vi "FGGA Serial Data Server & Recordingv4.2.vi"() -> ()   [LabVIEW 2014]
uses:
  <vilib>/Instr/_visa.llb/VISA Set IO Buffer Mask.ctl
  <vilib>/Instr/_visa.llb/VISA Flush IO Buffer Mask.ctl
  <vilib>/Platform/TimedLoop/XDataNode/timing_clust.ctl
  <vilib>/Platform/TimedLoop/XDataNode/nitl_modes.ctl
  <vilib>/Platform/TimedLoop/XDataNode/wakeup.ctl
  C:/Program Files (x86)/National Instruments/LabVIEW 2014/examples/Data Communication/Network Streams/Simple Network Streams/support/Network Stream Command.ctl
  <vilib>/Utility/error.llb/whitespace.ctl
  <vilib>/Instr/_visa.llb/VISA Configure Serial Port (Instr).vi
  <vilib>/Utility/tcp.llb/UDP Multicast Write-Only Open.vi
  <vilib>/platform/TimedLoop/XDataNode/XDataNode.xnode
  <vilib>/Platform/TimedLoop/XDataNode/XDNodeRunTimeDep.lvlib
panel:
  out "FGGA Pump":bool
  out "Flight Number":string
  out "Stop File Write":bool
  out "Default file name":string
  out "MFC":dbl[](array[numeric])
  out "FGGA restart":bool
  out "V4":bool
  out "V3":bool
  out "V2":bool
  out "V1":bool
  out "error out 2":errorcluster
  out "error out":errorcluster
  in  "MFC_1 SLPM set value":dbl
  out "Value Read":string
  out "status":bool
  in  "VISA resource name":refnum<visa-resource-name>="ASRL3::INSTR"
  in  "timeout (10sec) 2":u32=3000
  out "Labview_Viewer_UDP_Error_Out":errorcluster
  in  "Clear Display\nErrors":bool
  out "Data Processing":bool
  out "TCP Binary Packet":string
  out "UDP Time Stamp Offset":i32=1
  out "Data String":string
  out "UDP_ACSII_Out":string
  out "Serial error out":errorcluster
  out "SEPTIC TCP Error Out":errorcluster
  out "TCP packet\nSend To SEPTIC":bool
  out "FISH TCP Error Out":errorcluster
  out "TCP packet\nSend To FISH":bool
  out "UDP_Pack_num":u32
  out "UDP_Out Status":bool
  out "UDP_Out_Error Out":errorcluster
  out "Data Array":string[](array[string])
  out "RAW DATA":string
  in  "stop":bool
  in  "timeout (10sec)":u32=1500
  in  "VISA resource name":refnum<visa-resource-name>="ASRL7::INSTR"
  out "Number of times \nRead time out":u32
  out "Loop count":i32
  # "Date"
  # "Time"
  # "CH4"
  # "CO2"
  # "H2O"
  # "Cell Pressure"
  # "Cell Temperature"
  # "Spectral Flag"
  # "Ring Down Time (Laser A)"
  # "Ring Down Time (Laser B)"
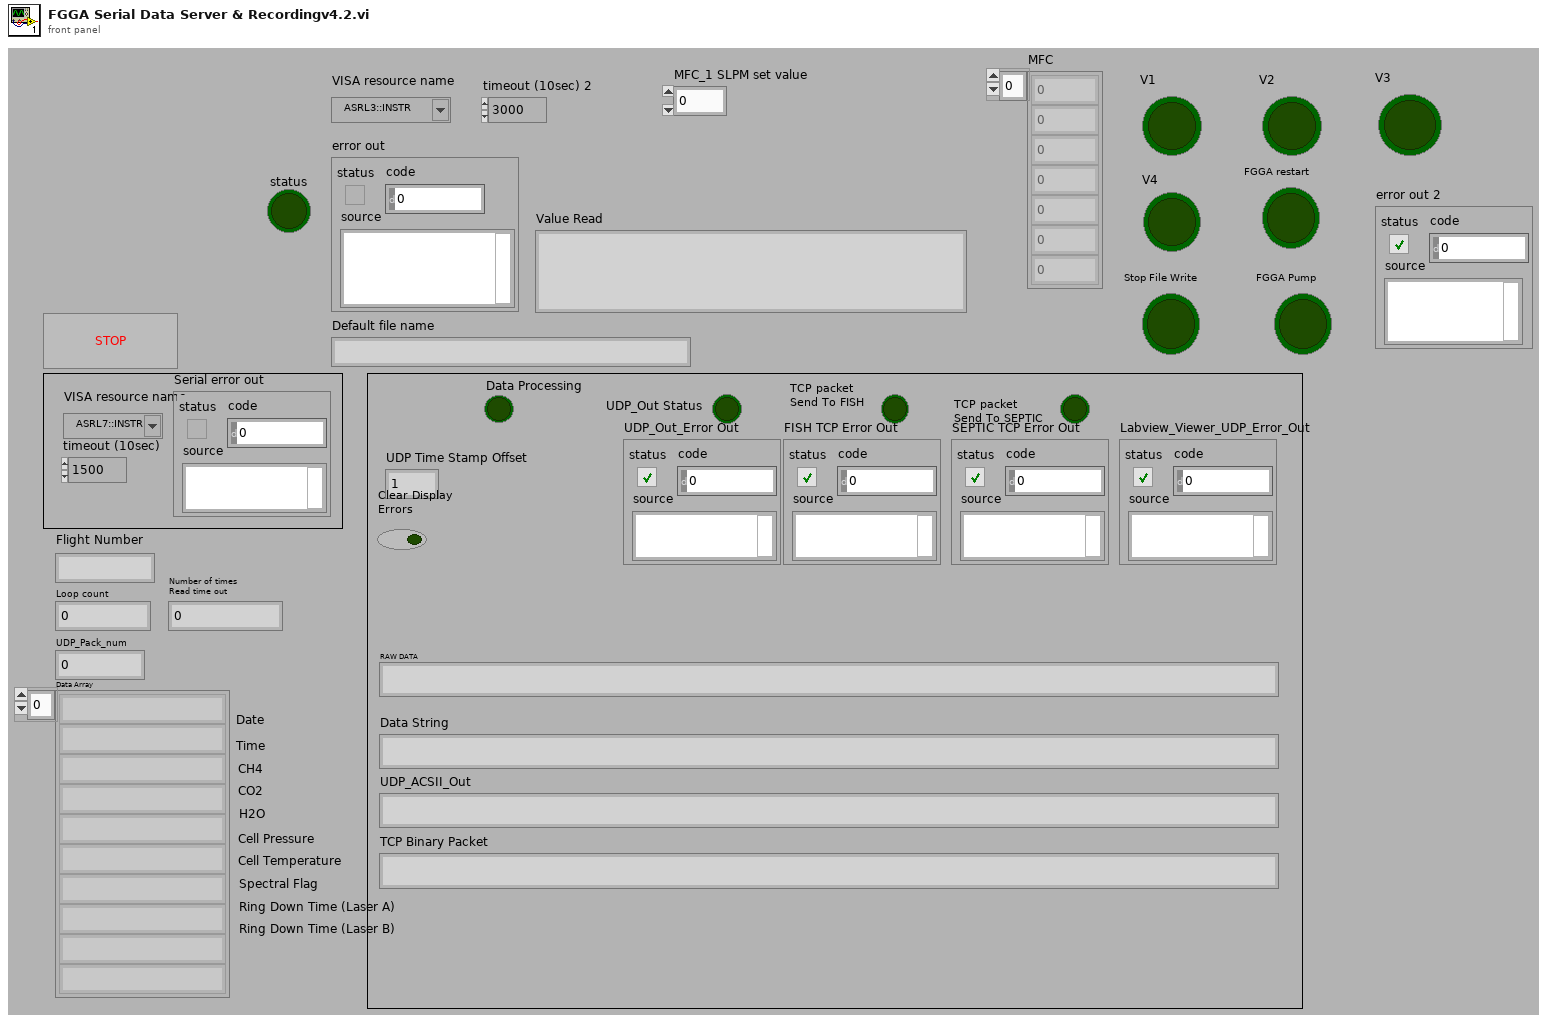
[diagram p1: front panel]
types:
  T1 = typedef "VISA Flush IO Buffer Mask.ctl" = u16
  T2 = typedef "VISA Set IO Buffer Mask.ctl" = u16
  T3 = typedef "XDNodeRunTimeDep.lvlib/timing_clust.ctl" = cluster{"Expected End [f-1]":u64, "Actual End [f-1]":u64, "Finished Late? [f-1]":bool, "Expected End [i-1]":u64, "Actual End [i-1]":u64, "Finished Late? [i-1]":bool, "Expected Start [i]":u64, "Actual Start [i]":u64, "Expected Start [f]":u64, "Actual Start [f]":u64, "Source Name":string, "Structure Name":string, "Period":i64, "Deadline":i64, "Offset":i64, "Start":i64, "Priority":i32, "Timeout":i32, "Mode":T4, "Wakeup Reason":T5, "Error":errorcluster, "Source Type":string, "Secondary Source Type":string, "Global End Time":u64, "Global Start Time":u64, "Frame Duration":u64, "Iteration Duration":u64, "Assigned CPU":i32, "I/O Scan Engine Mode":u32}
  T4 = typedef "XDNodeRunTimeDep.lvlib/nitl_modes.ctl" = enum32{"No Change", "Process missed periods, maintain original phase", "Discard missed periods, maintain original phase", "Process missed periods, ignore original phase", "Discard missed periods, ignore original phase"}
  T5 = typedef "XDNodeRunTimeDep.lvlib/wakeup.ctl" = enum32{"Normal", "Aborted", "Asynchronous wakeup", "Timing source error", "Timed loop error", "Timeout"}
  T6 = typedef "Network Stream Command.ctl" = cluster{"Message":string, "Message Data":variant}
  T7 = enum16{"open", "replace", "create", "open or create", "replace or create", "replace or create with confirmation"}
  T8 = typedef "whitespace.ctl" = u16
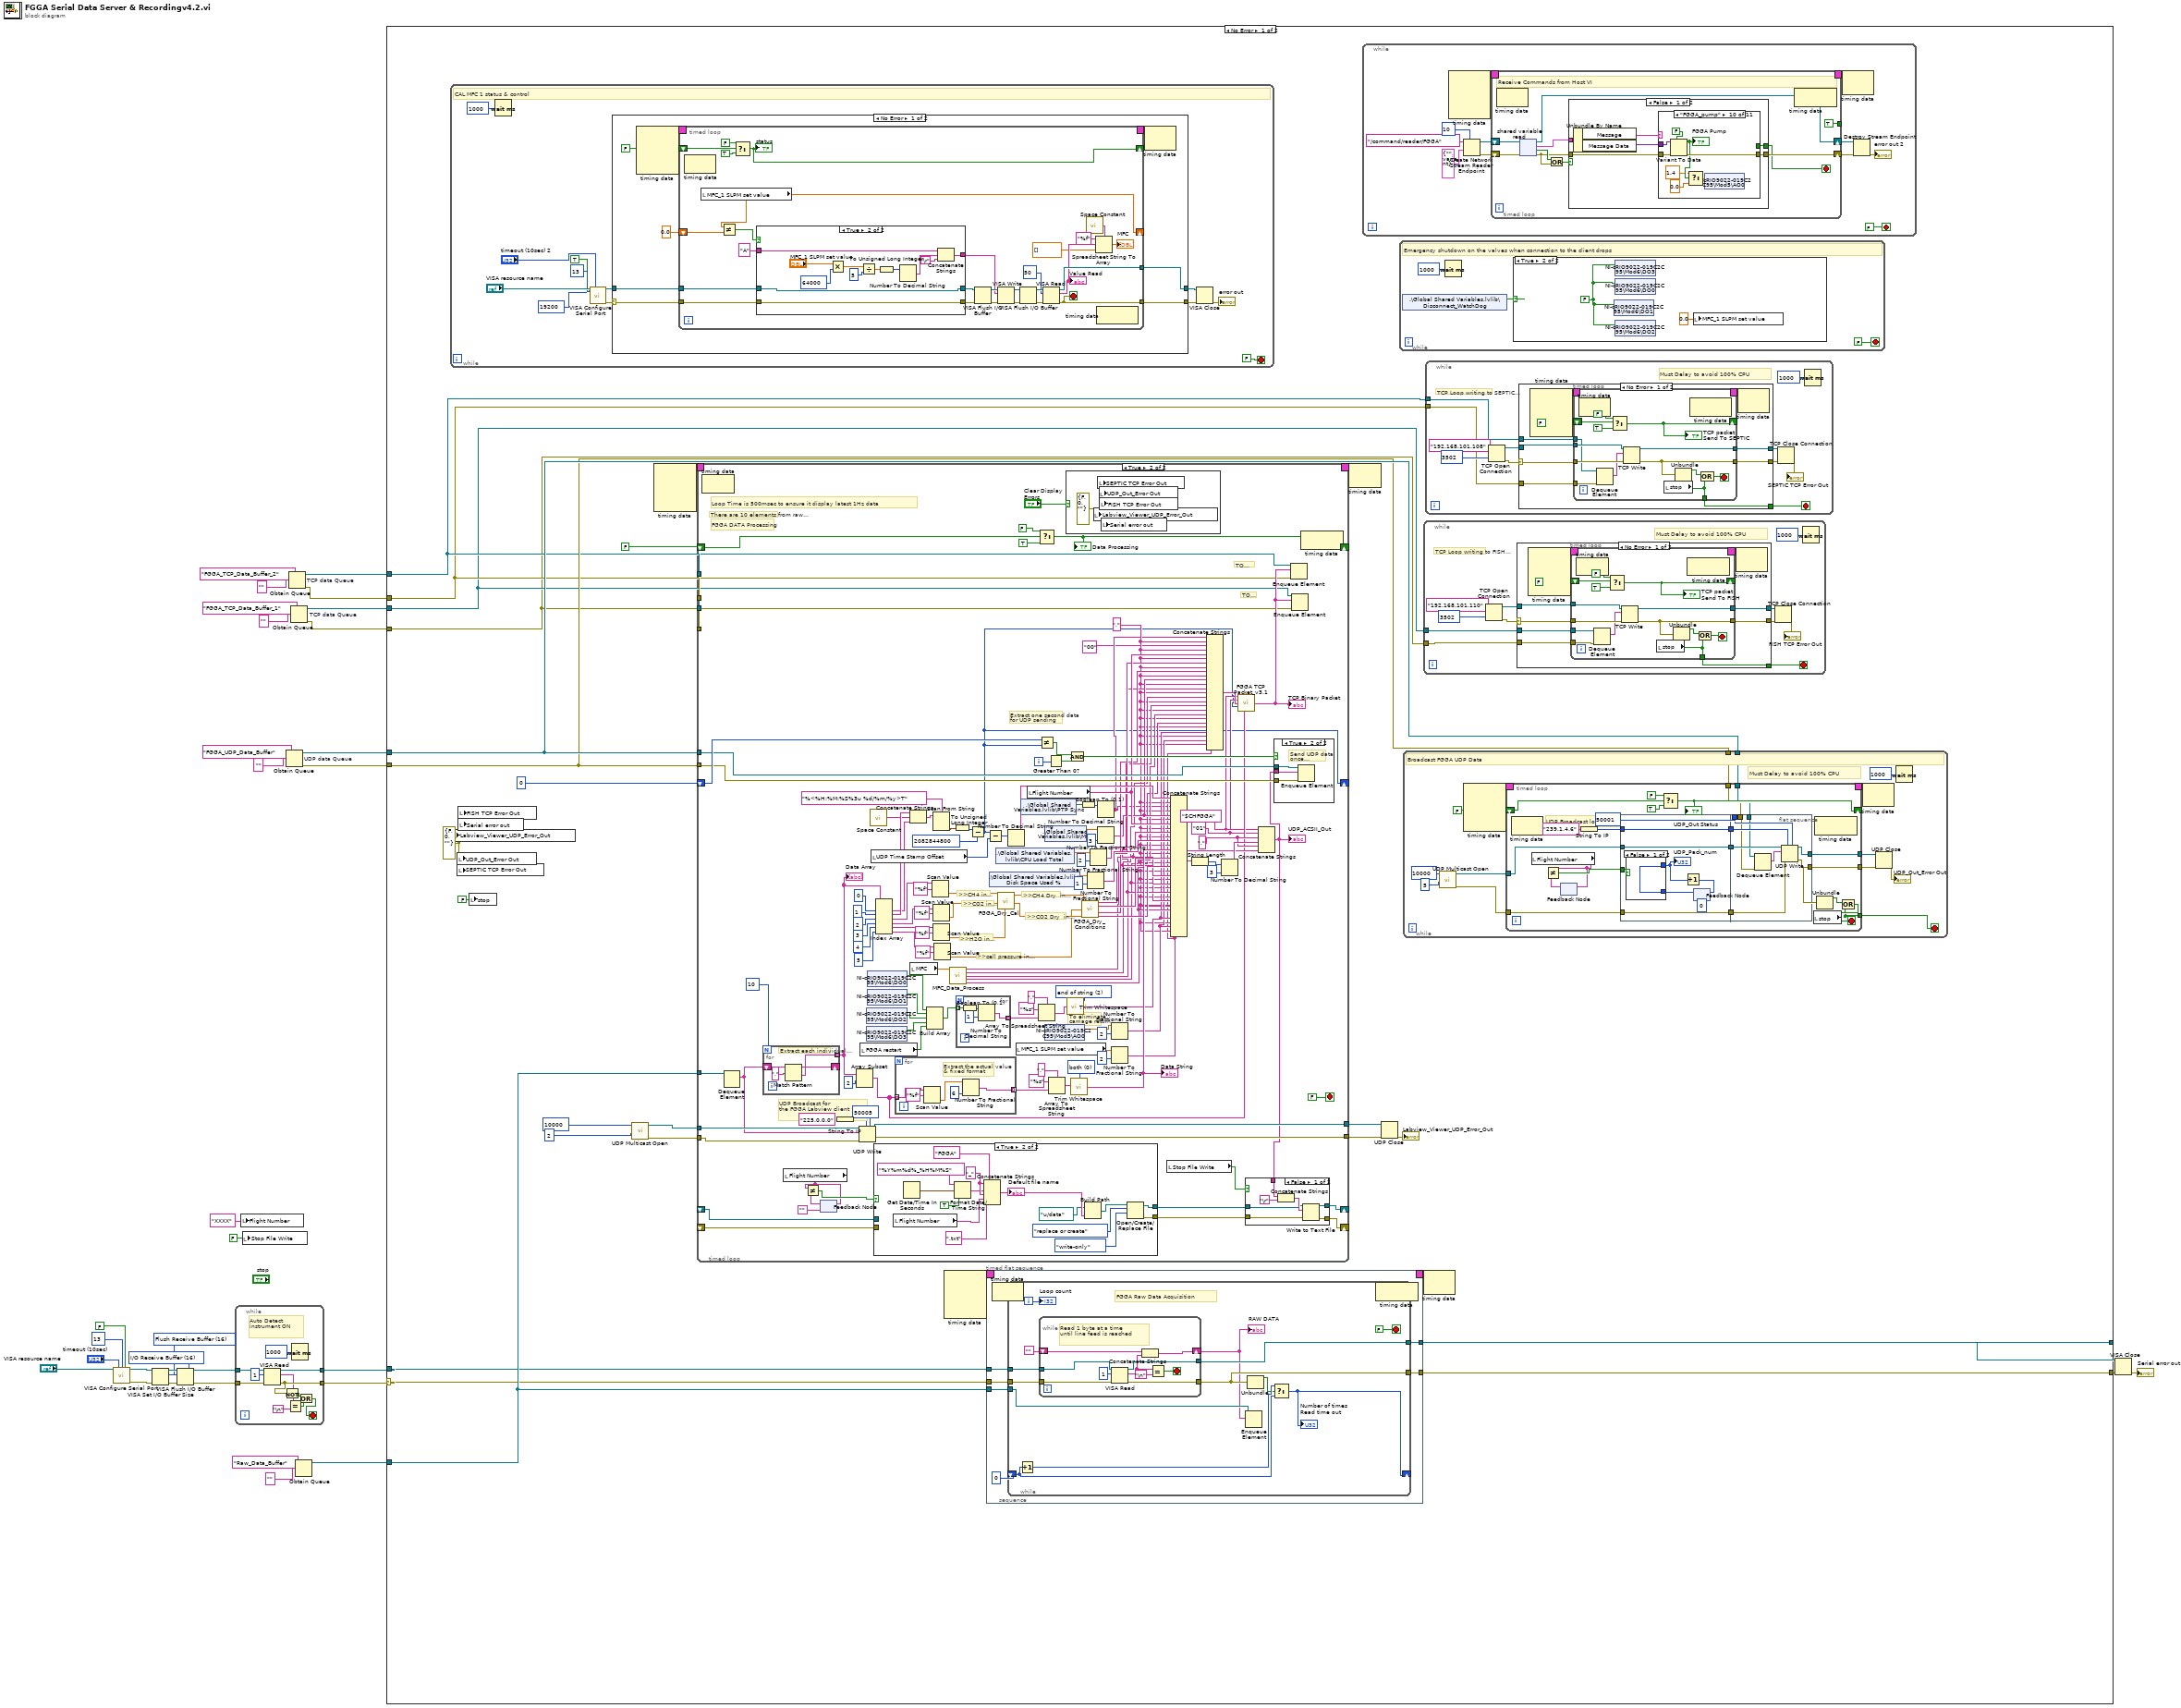
[diagram p0: block diagram]
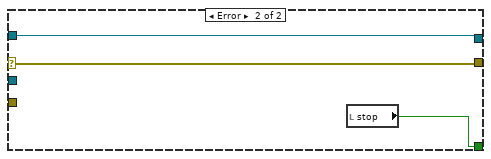
[diagram p3: hidden frame]
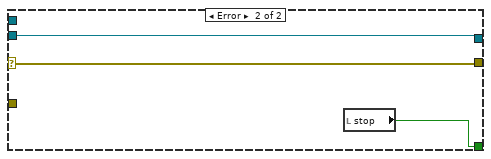
[diagram p4: hidden frame]
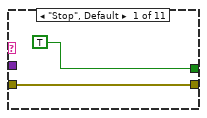
[diagram p5: hidden frame]
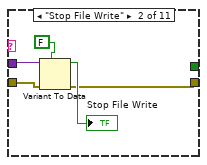
[diagram p6: hidden frame]
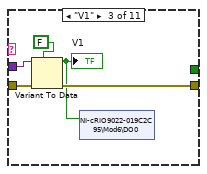
[diagram p7: hidden frame]
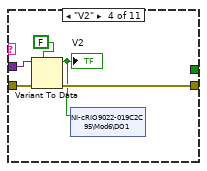
[diagram p8: hidden frame]
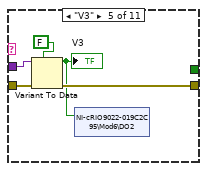
[diagram p9: hidden frame]
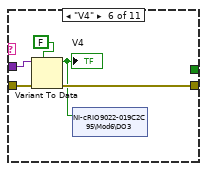
[diagram p10: hidden frame]
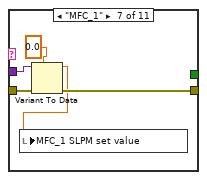
[diagram p11: hidden frame]
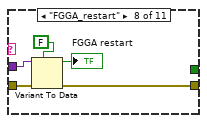
[diagram p12: hidden frame]
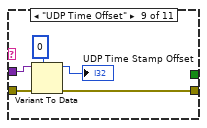
[diagram p13: hidden frame]
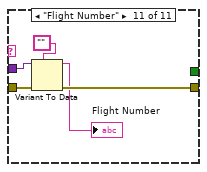
[diagram p14: hidden frame]
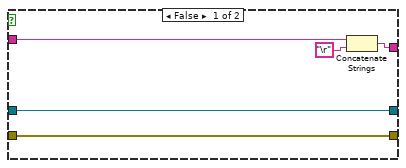
[diagram p16: hidden frame]
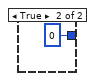
[diagram p18: hidden frame]
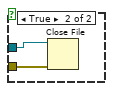
[diagram p20: hidden frame]
diagram:
  w9 = T1 16 items=["Flush Receive Buffer"=16, "Write Transmit Buffer to Device"=32, "Flush Receive Buffer (No I/O)"=64, "Flush Transmit Buffer"=128] ("Mask")
  w10 = T2 16 items=["I/O Receive Buffer"=16, "I/O Transmit Buffer"=32, "I/O Receive and Transmit Buffer"=48] ("Mask")
  n1 = call-poly "VISA Configure Serial Port"("VISA resource name"="VISA resource name", "timeout (10sec)"="timeout (10sec)", "termination char\n(0xA = '\\n' = LF)"=u8 13 ("termination char\n(0xA = '\\n' = LF)"), "Enable Termination\nChar (T)"=FALSE ("Enable Termination\nChar (T)")) -> ("VISA resource name out"=w8:refnum<visa-resource-name>, "error out"=w7:errorcluster)  [unwired: 10 in]
  n2 = VISA Set I/O Buffer Size(VISA resource name=w8, mask (16)=w10, error in (no error)=w7) -> (VISA resource name out=w11:refnum<visa-resource-name>, error out=w12:errorcluster)  [unwired: 1 in]
  n3 = VISA Flush I/O Buffer(VISA resource name=w11, mask (16)=w9, error in (no error)=w12) -> (VISA resource name out=w6:refnum<visa-resource-name>, error out=w5:errorcluster)
  n4 = while {
    tunnel: w6 -> [w45]
    tunnel: w5 -> [w44]
    tunnel: [w42] -> w4
    tunnel: [w41] -> w3
    stop <- w36 stop-if-true
    # "Auto Detect\ninstrument ON"
    n5 = VISA Read(VISA resource name=w45, byte count=u32 1, error in (no error)=w44) -> (VISA resource name out=w41:refnum<visa-resource-name>, read buffer=w39:string, error out=w42:errorcluster)  [unwired: 1 out]
    n6 = Not(x=w42) -> (.not. x?=w38:bool)
    n7 = Equal?(x=w39, y="\n") -> (x = y?=w37:bool)
    n8 = Wait (ms)(milliseconds to wait=u32 1000) -> ()  [unwired: 1 out]
    n9 = Or(x=w38, y=w37) -> (x .or. y?=w36:bool)
  }
  n10 = local write "Flight Number"("XXXX" ("Flight Number")) -> ()
  n11 = local write "Stop File Write"(FALSE ("Stop File Write")) -> ()
  n12 = Obtain Queue "UDP data Queue"(name (unnamed)="FGGA_UDP_Data_Buffer", element data type="") -> (queue out=w22:refnum<queue>, error out=w21:errorcluster)  [unwired: 3 in, 1 out]
  n13 = Obtain Queue "TCP data Queue"(name (unnamed)="FGGA_TCP_Data_Buffer_2", element data type="") -> (queue out=w16:refnum<queue>, error out=w15:errorcluster)  [unwired: 3 in, 1 out]
  n14 = Obtain Queue "TCP data Queue"(name (unnamed)="FGGA_TCP_Data_Buffer_1", element data type="") -> (queue out=w14:refnum<queue>, error out=w13:errorcluster)  [unwired: 3 in, 1 out]
  n15 = Obtain Queue(name (unnamed)="Raw_Data_Buffer", element data type="") -> (queue out=w28:refnum<queue>)  [unwired: 3 in, 2 out]
  n16 = case shown="No Error" w4 {
    selector: w4 -> [w48 w595]
    tunnel: w3 -> [w49 w596]
    tunnel: [w70 w596] -> w25
    tunnel: [w71 w595] -> w26
    tunnel: w28 -> [w67 _]
    tunnel: w22 -> [w65 _]
    tunnel: w21 -> [w64 _]
    tunnel: w16 -> [w63 _]
    tunnel: w15 -> [w62 _]
    tunnel: w14 -> [w61 _]
    tunnel: w13 -> [w60 _]
    frame No Error {
      w51 = errorcluster {"status"=FALSE, "code"=0, "source"=""} ("UDP Error Out")
      n17 = while {
        stop <- FALSE stop-if-true
        # "CAL MFC 1 status & control"
        n18 = Wait (ms)(milliseconds to wait=u32 1000) -> ()  [unwired: 1 out]
        n19 = call-poly "VISA Configure Serial Port"("VISA resource name"="VISA resource name", "timeout (10sec)"="timeout (10sec) 2", "termination char\n(0xA = '\\n' = LF)"=u8 13 ("termination char\n(0xA = '\\n' = LF)"), "Enable Termination\nChar (T)"=TRUE ("Enable Termination\nChar (T)"), "baud rate (9600)"=u32 19200) -> ("VISA resource name out"=w298:refnum<visa-resource-name>, "error out"=w294:errorcluster)  [unwired: 9 in]
        n20 = case shown="No Error" w294 {
          selector: w294 -> [w305 w355]
          tunnel: w298 -> [w306 w356]
          tunnel: [w304 w356] -> w297
          tunnel: [w303 w355] -> w296
          frame No Error {
            n21 = node-c288() -> (w301:T3)  [unwired: 4 in]
            n22 = timed-loop {
              tunnel: w306 -> [w329]
              tunnel: w305 -> [w327]
              tunnel: [w320] -> w304
              tunnel: [w315] -> w303
              shift-right: [w316] -> _
              shift-left: FALSE -> [w319]
              timing: w301 -> [_]
              timing-out: [_] -> w300
              shift-right: [w307] -> _
              shift-left: 0.0 -> [w309]
              stop <- w315 stop-if-true
              n23 = node-c288() -> ()  [unwired: 1 in, 1 out]
              n24 = local read "MFC_1 SLPM set value"() -> (w307:dbl)
              n25 = Not Equal?(x=w307, y=w309) -> (x != y?=w308:bool)
              n26 = Select(t=FALSE, s=w319, f=TRUE) -> (s? t:f=w316:bool)
              "status" <- w316
              n27 = case shown="True" w308 {
                tunnel: w329 -> [w337 w352]
                tunnel: [w337 w352] -> w328
                tunnel: w327 -> [w336 w351]
                tunnel: [w336 w351] -> w326
                tunnel: "A" -> [w340 w344]
                tunnel: [w338 w341] -> w324
                frame False {
                  n28 = Concatenate Strings(w340, "\r") -> (w338:string)
                }
                frame True {
                  n29 = Multiply(x="MFC_1 SLPM set value", y=u32 64000) -> (x*y=w348:dbl)
                  n30 = Divide(x=w348, y=u32 5) -> (x/y=w346:dbl)
                  n31 = To Unsigned Long Integer(number=w346) -> (unsigned 32bit integer=w345:u32)
                  n32 = Number To Decimal String(number=w345) -> (decimal integer string=w343:string)  [unwired: 1 in]
                  n33 = Concatenate Strings(w344, w343, "\r") -> (w341:string)
                }
              }
              n34 = VISA Flush I/O Buffer(VISA resource name=w328, error in (no error)=w326) -> (VISA resource name out=w331:refnum<visa-resource-name>, error out=w330:errorcluster)  [unwired: 1 in]
              n35 = VISA Write(VISA resource name=w331, write buffer=w324, error in (no error)=w330) -> (VISA resource name out=w323:refnum<visa-resource-name>, error out=w322:errorcluster)  [unwired: 1 out]
              n36 = VISA Flush I/O Buffer(VISA resource name=w323, error in (no error)=w322) -> (VISA resource name out=w333:refnum<visa-resource-name>, error out=w332:errorcluster)  [unwired: 1 in]
              n37 = VISA Read(VISA resource name=w333, byte count=u32 50, error in (no error)=w332) -> (VISA resource name out=w320:refnum<visa-resource-name>, read buffer=w314:string, error out=w315:errorcluster)  [unwired: 1 out]
              "Value Read" <- w314
              n38 = call <vilib>:"Space Constant.vi"() -> ("String"=w313:string)
              n39 = Spreadsheet String To Array(delimiter (Tab)=w313, format string="%f", spreadsheet string=w314, array type (2D Dbl)=dbl[] []) -> (array=→"MFC":dbl[])
              n40 = node-c288() -> ()  [unwired: 1 in, 1 out]
            }
            n41 = node-c288(w300) -> ()  [unwired: 1 out]
          }
          frame Error {
          }
        }
        n42 = VISA Close(VISA resource name=w297, error in (no error)=w296) -> (error out=→"error out":errorcluster)
      }
      n43 = local write "Labview_Viewer_UDP_Error_Out"(w51) -> ()
      n44 = local write "UDP_Out_Error Out"(w51) -> ()
      n45 = local write "SEPTIC TCP Error Out"(w51) -> ()
      n46 = local write "FISH TCP Error Out"(w51) -> ()
      n47 = local write "Serial error out"(w51) -> ()
      n48 = local write "stop"(FALSE ("stop")) -> ()
      n49 = call-poly <vilib>:"UDP Multicast Open.vi"("time-to-live (1)"=u16 2, "port"=u16 10000) -> ("error out"=w55:errorcluster, "connection ID"=w56:refnum<k16>)  [unwired: 8 in]
      n50 = node-c288() -> (w69:T3)  [unwired: 4 in]
      n51 = timed-loop {
        timing: w69 -> [_]
        timing-out: [_] -> w68
        tunnel: w67 -> [w547]
        tunnel: w65 -> [w503]
        tunnel: w64 -> [w502]
        shift-right: [w416] -> _
        shift-left: u32 0 -> [w506]
        tunnel: w63 -> [w499]
        tunnel: w62 -> [w498]
        tunnel: w61 -> [w497]
        tunnel: w60 -> [w496]
        shift-right: [w492] -> _
        shift-left: FALSE -> [w495]
        tunnel: w56 -> [w488]
        tunnel: w55 -> [w487]
        tunnel: [w486] -> w54
        tunnel: [w485] -> w53
        shift-right: [w472] -> _
        shift-left: _ -> [w464]
        shift-right: [w462] -> _
        shift-left: _ -> [w463]
        i -> [w505]
        stop <- FALSE stop-if-true
        w436 = T8 2 items=["both", "start of string", "end of string"] ("location (both)")
        w423 = ","
        w533 = T8 0 items=["both", "start of string", "end of string"] ("location (both)")
        w541 = ","
        w417 = "01"
        w418 = "$CHFGGA"
        # "To eliminate\ncarriage return"
        # ">>cell pressure in torr>>"
        # "UDP Broadcast for\nthe FGGA Labview client"
        # "There are 10 elements from raw packet"
        # "TO SEPTIC"
        # "TO FISH"
        # "Extract one second data\nfor UDP sending"
        # ">>CO2 Dry  in ppm>>"
        # ">>CH4 Dry  in ppb>>"
        # ">>H2O in ppm>>"
        # ">>CO2 in ppm>>"
        # ">>CH4 in ppm>>"
        # "Loop Time is 500msec to ensure it display latest 1Hz data"
        # "FGGA DATA Processing"
        n52 = node-c288() -> ()  [unwired: 1 in, 1 out]
        n53 = Dequeue Element(queue=w547) -> (element=w484:string)  [unwired: 2 in, 3 out]
        n54 = for {
          N: 10 -> [_]
          shift-right: [w589] -> _
          shift-left: w484 -> [w587]
          tunnel: [w588] -> w538 mode=indexing
          # "Extract each individual param"
          n55 = Match Pattern(string=w587, regular expression=",") -> (before substring=w588:string, after substring=w589:string)  [unwired: 1 in, 2 out]
        }
        "Data Array" <- w538
        n56 = local read "Flight Number"() -> (w461:string)
        n57 = feedback #1("" ("Flight Number")) -> (w469:string)
        n58 = Not Equal?(x=w461, y=w469) -> (x != y?=w467:bool)
        n59 = feedback-in #1(w461) -> ()
        n60 = String To IP(1:"225.0.0.0" ("name")) -> (0:w489:u32)
        n61 = Array Subset(array=w538, index=2) -> (w501:string[])  [unwired: 1 in]
        n62 = UDP Write(address=w489, port or service name=u16 50005, connection ID=w488, data in=w484, 8:w487) -> (error out=w485:errorcluster, 3:w486:refnum<k16>)  [unwired: 1 in]
        n63 = local read "FGGA restart"() -> (w446:bool)
        n64 = shared-variable "NI-cRIO9022-019C2C95\\Mod6\\DO2"() -> (w452:bool)  [unwired: 1 in, 1 out]
        n65 = shared-variable "NI-cRIO9022-019C2C95\\Mod6\\DO3"() -> (w451:bool)  [unwired: 1 in, 1 out]
        n66 = shared-variable "NI-cRIO9022-019C2C95\\Mod6\\DO0"() -> (w454:bool)  [unwired: 1 in, 1 out]
        n67 = shared-variable "NI-cRIO9022-019C2C95\\Mod6\\DO1"() -> (w453:bool)  [unwired: 1 in, 1 out]
        n68 = call <vilib>:"Space Constant.vi"() -> ("String"=w516:string)
        n69 = local read "UDP Time Stamp Offset"() -> (w435:i32)
        n70 = case shown="True" w467 {
          tunnel: [w553 w555] -> w466
          tunnel: [w552 w554] -> w465
          tunnel: w464 -> [w553 _]
          tunnel: w463 -> [w552 _]
          frame False {
          }
          frame True {
            w561 = "_" ("string")
            n71 = local read "Flight Number"() -> (w568:string)
            n72 = Get Date/Time In Seconds() -> (seconds since 1Jan1904=w556:timestamp)
            n73 = Format Date/Time String(time format string (%c)="%Y%m%d%_%H%M%S", seconds (now)=w556, UTC format=TRUE) -> (date/time string=w558:string)
            n74 = Concatenate Strings("FGGA" ("string"), w561, w558, w561, w568, ".txt" ("string")) -> (w563:string)
            "Default file name" <- w563
            n75 = Build Path(base path=path "u:/data", name or relative path=w563) -> (appended path=w567:path)
            n76 = Open/Create/Replace File(file path (use dialog)=w567, operation (0:open)=T7."replace or create", access (0:read/write)=enum16{"read/write", "read-only", "write-only"}."write-only") -> (refnum out=w555:refnum<file>, error out=w554:errorcluster)  [unwired: 3 in, 1 out]
          }
        }
        n77 = Index Array(array=w538, index #1=0 ("index"), index #2=1 ("index"), index #3=2 ("index"), index #4=3 ("index"), index #5=4 ("index"), index #6=5 ("index")) -> (element #1=w515:string, element #2=w517:string, element #3=w521:string, element #4=w520:string, element #5=w519:string, element #6=w477:string)
        n78 = for {
          tunnel: w501 -> [w585] mode=indexing
          tunnel: [w582] -> w531 mode=indexing
          # "Extract the actual value\n& fixed format"
          n79 = Scan Value(string=w585, format string="%f") -> (value=w583:dbl)  [unwired: 1 in, 1 out]
          n80 = Number To Fractional String(number=w583, precision (6)=i16 6) -> (F-format string=w582:string)  [unwired: 2 in]
        }
        n81 = Concatenate Strings(w517, w516, w515) -> (w514:string)
        n82 = local read "MFC"() -> (w473:dbl[])
        n83 = Build Array(w454, w453, w452, w451, w446) -> (w450:bool[])
        n84 = Scan Value(string=w521, format string="%f") -> (value=w523:dbl)  [unwired: 1 in, 1 out]
        n85 = Scan Value(string=w520, format string="%f") -> (value=w522:dbl)  [unwired: 1 in, 1 out]
        n86 = Scan From String(format string="%<%H:%M:%S%3u %d/%m/%y>T", input string=w514) -> (output 1=w511:timestamp)  [unwired: 3 in, 3 out]
        n87 = Scan Value(string=w519, format string="%f") -> (value=w474:dbl)  [unwired: 1 in, 1 out]
        n88 = Scan Value(string=w477, format string="%f") -> (value=w475:dbl)  [unwired: 1 in, 1 out]
        n89 = call "MFC_Data_Process.vi"("MFC"=w473) -> ("MFC Absolute Pressure"=w430:string, "MFC Temperature"=w429:string, "MFC Volumetric Flow"=w428:string, "MFC Mass Flow"=w427:string, "MFC Set Point"=w426:string)  [unwired: 10 in]
        n90 = To Unsigned Long Integer(number=w511) -> (unsigned 32bit integer=w512:u32)
        n91 = for {
          tunnel: w450 -> [w550] mode=indexing
          tunnel: [w549] -> w447 mode=indexing
          n92 = Boolean To (0,1)(Boolean=w550) -> (0, 1=w551:i16)
          n93 = Number To Decimal String(number=w551, width (-)=i16 1) -> (decimal integer string=w549:string)
        }
        n94 = Subtract(x=w512, y=u32 2082844800) -> (x-y=w416:u32)
        n95 = Subtract(x=w416, y=w435) -> (x-y=w509:u32)
        n96 = shared-variable ".\\Global Shared Variables.lvlib\\Disk Space Used %"() -> (w439:dbl)  [unwired: 1 in, 1 out]
        n97 = shared-variable ".\\Global Shared Variables.lvlib\\CPU Load Total"() -> (w460:dbl)  [unwired: 1 in, 1 out]
        n98 = call "FGGA_Dry_Cal.vi"("H2O"=w474, "CO2_Wet"=w522, "CH4_Wet"=w523) -> ("CO2_Dry"=w479:dbl, "CH4_Dry"=w481:dbl)  [unwired: 7 in]
        n99 = Number To Decimal String(number=w509) -> (decimal integer string=w510:string)  [unwired: 1 in]
        n100 = local read "MFC_1 SLPM set value"() -> (w442:dbl)
        n101 = shared-variable ".\\Global Shared Variables.lvlib\\PTP Sync"() -> (w455:bool)  [unwired: 1 in, 1 out]
        n102 = local read "Flight Number"() -> (w434:string)
        n103 = Array To Spreadsheet String(delimiter (Tab)=",", array=w447, 3:"%s" ("format string")) -> (spreadsheet string=w437:string)
        n104 = Select(t=FALSE, s=w495, f=TRUE) -> (s? t:f=w492:bool)
        "Data Processing" <- w492
        n105 = Not Equal?(x=w506, y=w416) -> (x != y?=w507:bool)
        n106 = shared-variable ".\\Global Shared Variables.lvlib\\MFM"() -> (w458:dbl)  [unwired: 1 in, 1 out]
        n107 = shared-variable "NI-cRIO9022-019C2C95\\Mod5\\AO0"() -> (w444:dbl)  [unwired: 1 in, 1 out]
        n108 = Greater Than 0?(x=w505) -> (x > 0?=w508:bool)
        n109 = Array To Spreadsheet String(delimiter (Tab)=",", array=w531, 3:"%s" ("format string")) -> (spreadsheet string=w532:string)
        n110 = case shown="True" "Clear Display\nErrors" {
          frame False {
          }
          frame True {
            w578 = errorcluster {"status"=FALSE, "code"=0, "source"=""} ("UDP Error Out")
            n111 = local write "Labview_Viewer_UDP_Error_Out"(w578) -> ()
            n112 = local write "SEPTIC TCP Error Out"(w578) -> ()
            n113 = local write "UDP_Out_Error Out"(w578) -> ()
            n114 = local write "FISH TCP Error Out"(w578) -> ()
            n115 = local write "Serial error out"(w578) -> ()
          }
        }
        n116 = call <vilib>:"Trim Whitespace.vi"("string"=w437, "location (both)"=w436) -> ("trimmed string"=w425:string)
        n117 = call <vilib>:"Trim Whitespace.vi"("string"=w532, "location (both)"=w533) -> ("trimmed string"=w530:string)
        "Data String" <- w530
        n118 = Compound Arithmetic op=AND(w507, w508) -> (w504:bool)
        n119 = Boolean To (0,1)(Boolean=w455) -> (0, 1=w456:i16)
        n120 = call "FGGA_Dry_Conditions.vi"("CH4_Dry"=w481, "Pressure"=w475, "CO2_Dry"=w479) -> ("CH4_Dry_TCP"=w433:string, "CH4_Dry_UDP"=w483:string, "CO2_Dry_TCP"=w432:string, "CO2_Dry_UDP"=w482:string)  [unwired: 9 in]
        n121 = Number To Fractional String(number=w439, precision (6)=i16 1) -> (F-format string=w438:string)  [unwired: 2 in]
        n122 = Number To Fractional String(number=w460, precision (6)=i16 2) -> (F-format string=w441:string)  [unwired: 2 in]
        n123 = Number To Decimal String(number=w456) -> (decimal integer string=w420:string)  [unwired: 1 in]
        n124 = Number To Fractional String(number=w458, precision (6)=i16 3) -> (F-format string=w431:string)  [unwired: 2 in]
        n125 = Number To Fractional String(number=w444, precision (6)=i16 2) -> (F-format string=w424:string)  [unwired: 2 in]
        n126 = Number To Fractional String(number=w442, precision (6)=i16 2) -> (F-format string=w422:string)  [unwired: 2 in]
        n127 = local read "Stop File Write"() -> (w470:bool)
        n128 = Concatenate Strings(w510, w423, w420, w423, w431, w423, w434, w423, w441, w423, w438, w423, w530, w423, w483, w423, w482, w423, w430, w423, w429, w423, w428, w423, w427, w423, w426, w423, w425, w423, w424, w423, w422) -> (w540:string)
        n129 = String Length(string=w540) -> (length=w544:i32)
        n130 = Concatenate Strings(w420, w423, "00", w423, w434, w423, w433, w423, w432, w423, w431, w423, w430, w423, w429, w423, w428, w423, w427, w423, w426, w423, w425, w423, w424, w423, w422) -> (w421:string)
        n131 = Number To Decimal String(number=w544, width (-)=i16 3) -> (decimal integer string=w542:string)
        n132 = call "FGGA TCP Packet_v3.1.vi"("ID"=w418, "Version"=w417, "TCP Packet In"=w421, "utc_time"=w416, "Data Array"=w501) -> ("TCP Binary Packet"=w500:string)  [unwired: 10 in]
        "TCP Binary Packet" <- w500
        n133 = Concatenate Strings(w418, w417, w541, w542, w541, w540) -> (w471:string)
        "UDP_ACSII_Out" <- w471
        n134 = case shown="False" w470 {
          tunnel: w471 -> [w575 _]
          tunnel: [w572 _] -> w472
          tunnel: w466 -> [w571 w577]
          tunnel: w465 -> [w570 w576]
          tunnel: [w569 _] -> w462
          frame False {
            n135 = Concatenate Strings(w575, "\r") -> (w573:string)
            n136 = Write to Text File(file (use dialog)=w571, text=w573, error in=w570) -> (refnum out=w572:refnum<file>, error out=w569:errorcluster)  [unwired: 2 out]
          }
          frame True {
            n137 = Close File(refnum=w577, error in=w576) -> ()  [unwired: 2 out]
          }
        }
        n138 = case shown="True" w504 {
          tunnel: w471 -> [_ w581]
          tunnel: w503 -> [_ w580]
          tunnel: w502 -> [_ w579]
          frame False {
          }
          frame True {
            # "Send UDP data once\na second"
            n139 = Enqueue Element(queue=w580, element=w581, error in (no error)=w579) -> ()  [unwired: 1 in, 3 out]
          }
        }
        n140 = Enqueue Element(queue=w499, element=w500, error in (no error)=w498) -> ()  [unwired: 1 in, 3 out]
        n141 = Enqueue Element(queue=w497, element=w500, error in (no error)=w496) -> ()  [unwired: 1 in, 3 out]
        n142 = node-c288() -> ()  [unwired: 1 in, 1 out]
      }
      n143 = node-c288() -> (w47:T3)  [unwired: 4 in]
      n144 = timed-sequence {
        timing: w47 -> [_]
        timing-out: [_] -> w46
        tunnel: [w165] -> w71
        tunnel: [w164] -> w70
        tunnel: w67 -> [w163]
        tunnel: w49 -> [w162]
        tunnel: w48 -> [w161]
        n145 = timed-flat-sequence {
          tunnel: [w171] -> w165
          tunnel: [w170] -> w164
          tunnel: w163 -> [w168]
          tunnel: w162 -> [w167]
          tunnel: w161 -> [w166]
          n146 = node-c288() -> ()  [unwired: 1 in, 1 out]
          n147 = while {
            tunnel: w167 -> [w184]
            tunnel: w166 -> [w183]
            tunnel: [w182] -> w171
            shift-right: [w178] -> _
            shift-left: u32 0 -> [w179]
            tunnel: [w181] -> w170
            tunnel: w168 -> [w175]
            i -> [w180]
            stop <- FALSE stop-if-true
            # "FGGA Raw Data Acquisition"
            n148 = Increment(x=w179) -> (x+1=w177:u32)
            n149 = while {
              tunnel: [w194] -> w181
              tunnel: [w193] -> w182
              tunnel: w184 -> [w192]
              tunnel: w183 -> [w191]
              shift-right: [w189] -> w174
              shift-left: "" -> [w190]
              stop <- w186 stop-if-true
              # "Read 1 byte at a time \nuntil line feed is reached"
              n150 = VISA Read(VISA resource name=w192, byte count=u32 1, error in (no error)=w191) -> (VISA resource name out=w194:refnum<visa-resource-name>, read buffer=w188:string, error out=w193:errorcluster)  [unwired: 1 out]
              n151 = Concatenate Strings(w190, w188) -> (w189:string)
              n152 = Equal?(x=w188, y="\n") -> (x = y?=w186:bool)
            }
            "RAW DATA" <- w174
            n153 = Enqueue Element(queue=w175, element=w174) -> ()  [unwired: 2 in, 3 out]
            n154 = Unbundle(w182) -> ("status"=w173:bool)  [unwired: 2 out]
            n155 = Select(t=w177, s=w173, f=w179) -> (s? t:f=w178:u32)
            "Number of times \nRead time out" <- w178
            "Loop count" <- w180
          }
          n156 = node-c288() -> ()  [unwired: 1 in, 1 out]
        }
      }
      n157 = node-c288(w68) -> ()  [unwired: 1 out]
      n158 = while {
        stop <- FALSE stop-if-true
        n159 = node-c288() -> (w200:T3)  [unwired: 4 in]
        n160 = Create Network Stream Reader Endpoint(7:10 ("reader buffer size"), 9:T6 {"Message"="", "Message Data"=variant} ("Message Cluster"), 11:"/command/reader/FGGA" ("reader url")) -> (0:w205:errorcluster, 3:w206:refnum<k21>)  [unwired: 4 in]
        n161 = timed-loop "Host->Target Command Reader" {
          shift-right: [w216] -> w203
          shift-left: w205 -> [w219]
          shift-right: [w217] -> w202
          shift-left: w206 -> [w218]
          tunnel: [TRUE] -> _
          timing: w200 -> [_]
          timing-out: [_] -> w199
          stop <- w210 stop-if-true
          # "Receive Commands from Host VI"
          n162 = node-c288() -> ()  [unwired: 1 in, 1 out]
          n163 = shared-variable-read(w218, w219) -> (w217:refnum<k21>, w212:errorcluster, w214:bool, w215:T6)  [unwired: 1 in]
          n164 = Or(x=w214, y=w212) -> (x .or. y?=w213:bool)
          n165 = case shown="False" w213 {
            selector: w213 -> [_ w283]
            tunnel: w212 -> [w227 w284]
            tunnel: [w226 w284] -> w216
            tunnel: w215 -> [w224 _]
            tunnel: [w225 w283] -> w210
            frame False {
              n166 = Unbundle By Name(w224) -> ("Message"=w223:string, "Message Data"=w222:variant)
              n167 = case shown="\"FGGA_pump\"" w223 {
                tunnel: w227 -> [w229 w234 w239 w244 w249 w254 w259 w264 w269 w277 w282]
                tunnel: [w229 w230 w238 w243 w248 w253 w258 w263 w268 w276 w281] -> w226
                tunnel: w222 -> [_ w233 w237 w242 w247 w252 w257 w262 w267 w275 w280]
                tunnel: [TRUE _ _ _ _ _ _ _ _ _ _] -> w225
                frame "Stop", Default {
                }
                frame "Stop File Write" {
                  n168 = Variant To Data(error in=w234, type=FALSE, Variant=w233) -> (data=→"Stop File Write":bool, error out=w230:errorcluster)
                }
                frame "V1" {
                  n169 = Variant To Data(error in=w239, type=FALSE, Variant=w237) -> (data=w235:bool, error out=w238:errorcluster)
                  "V1" <- w235
                  n170 = shared-variable "NI-cRIO9022-019C2C95\\Mod6\\DO0"(w235) -> ()  [unwired: 1 in, 1 out]
                }
                frame "V2" {
                  n171 = Variant To Data(error in=w244, type=FALSE, Variant=w242) -> (data=w240:bool, error out=w243:errorcluster)
                  "V2" <- w240
                  n172 = shared-variable "NI-cRIO9022-019C2C95\\Mod6\\DO1"(w240) -> ()  [unwired: 1 in, 1 out]
                }
                frame "V3" {
                  n173 = Variant To Data(error in=w249, type=FALSE, Variant=w247) -> (data=w245:bool, error out=w248:errorcluster)
                  "V3" <- w245
                  n174 = shared-variable "NI-cRIO9022-019C2C95\\Mod6\\DO2"(w245) -> ()  [unwired: 1 in, 1 out]
                }
                frame "V4" {
                  n175 = Variant To Data(error in=w254, type=FALSE, Variant=w252) -> (data=w250:bool, error out=w253:errorcluster)
                  "V4" <- w250
                  n176 = shared-variable "NI-cRIO9022-019C2C95\\Mod6\\DO3"(w250) -> ()  [unwired: 1 in, 1 out]
                }
                frame "MFC_1" {
                  n177 = Variant To Data(error in=w259, type=0.0, Variant=w257) -> (data=w255:dbl, error out=w258:errorcluster)
                  n178 = local write "MFC_1 SLPM set value"(w255) -> ()
                }
                frame "FGGA_restart" {
                  n179 = Variant To Data(error in=w264, type=FALSE, Variant=w262) -> (data=→"FGGA restart":bool, error out=w263:errorcluster)
                }
                frame "UDP Time Offset" {
                  n180 = Variant To Data(error in=w269, type=0, Variant=w267) -> (data=→"UDP Time Stamp Offset":i32, error out=w268:errorcluster)
                }
                frame "FGGA_pump" {
                  n181 = Variant To Data(error in=w277, type=FALSE, Variant=w275) -> (data=w272:bool, error out=w276:errorcluster)
                  "FGGA Pump" <- w272
                  n182 = Select(t=1.4 ("f"), s=w272, f=0.0 ("t")) -> (s? t:f=w273:dbl)
                  n183 = shared-variable "NI-cRIO9022-019C2C95\\Mod5\\AO0"(w273) -> ()  [unwired: 1 in, 1 out]
                }
                frame "Flight Number" {
                  n184 = Variant To Data(error in=w282, type="", Variant=w280) -> (data=→"Flight Number":string, error out=w281:errorcluster)
                }
              }
            }
            frame True {
            }
          }
          n185 = node-c288() -> ()  [unwired: 1 in, 1 out]
        }
        n186 = node-c288(w199) -> ()  [unwired: 1 out]
        n187 = Destroy Stream Endpoint(8:w203, 11:w202) -> (0:→"error out 2":errorcluster)
      }
      n188 = UDP Close(connection ID=w54, 8:w53) -> (error out=→"Labview_Viewer_UDP_Error_Out":errorcluster)  [unwired: 1 out]
      n189 = while {
        stop <- FALSE stop-if-true
        # "Emergency shutdown on the valves when connection to the client drops"
        n190 = shared-variable ".\\Global Shared Variables.lvlib\\Disconnect_WatchDog"() -> (w72:bool)  [unwired: 1 in, 1 out]
        n191 = Wait (ms)(milliseconds to wait=u32 1000) -> ()  [unwired: 1 out]
        n192 = case shown="True" w72 {
          frame False {
          }
          frame True {
            w76 = FALSE
            n193 = shared-variable "NI-cRIO9022-019C2C95\\Mod6\\DO1"(w76) -> ()  [unwired: 1 in, 1 out]
            n194 = shared-variable "NI-cRIO9022-019C2C95\\Mod6\\DO3"(w76) -> ()  [unwired: 1 in, 1 out]
            n195 = shared-variable "NI-cRIO9022-019C2C95\\Mod6\\DO0"(w76) -> ()  [unwired: 1 in, 1 out]
            n196 = shared-variable "NI-cRIO9022-019C2C95\\Mod6\\DO2"(w76) -> ()  [unwired: 1 in, 1 out]
            n197 = local write "MFC_1 SLPM set value"(0.0 ("MFC_1 SLPM set value")) -> ()
          }
        }
      }
      n198 = while {
        tunnel: w65 -> [w359]
        tunnel: w64 -> [w358]
        stop <- w360 stop-if-true
        # "Must Delay to avoid 100% CPU"
        # "Broadcast FGGA UDP Data"
        n199 = call-poly <vilib>:"UDP Multicast Open.vi"("time-to-live (1)"=u16 5, "port"=u16 10000) -> ("error out"=w367:errorcluster, "connection ID"=w368:refnum<k16>)  [unwired: 8 in]
        n200 = node-c288() -> (w370:T3)  [unwired: 4 in]
        n201 = timed-loop {
          tunnel: w368 -> [w391]
          tunnel: w367 -> [w390]
          timing: w370 -> [_]
          timing-out: [_] -> w369
          shift-right: [w379] -> _
          shift-left: FALSE -> [w382]
          tunnel: [w378] -> w362
          tunnel: [w376] -> w361
          tunnel: [w374] -> w360
          tunnel: w359 -> [w372]
          tunnel: w358 -> [w371]
          stop <- w375 stop-if-true
          # "UDP Broadcast loop"
          n202 = node-c288() -> ()  [unwired: 1 in, 1 out]
          n203 = local read "Flight Number"() -> (w373:string)
          n204 = feedback-in #2(w373) -> ()
          n205 = feedback #2() -> (w384:string)  [unwired: 1 in]
          n206 = Not Equal?(x=w373, y=w384) -> (x != y?=w383:bool)
          n207 = String To IP(1:"239.1.4.6" ("name")) -> (0:w388:u32)
          n208 = flat-sequence {
            tunnel: w388 -> [w398]
            tunnel: w390 -> [w399]
            tunnel: w391 -> [w400]
            tunnel: [w400] -> w387
            tunnel: [w399] -> w386
            tunnel: [w398] -> w385
            tunnel: w383 -> [w397]
            tunnel: u16 50001 ("port or service name") -> [w411]
            tunnel: w387 -> [w410]
            tunnel: w386 -> [w409]
            tunnel: w385 -> [w408]
            tunnel: [w407] -> w378
            tunnel: [w406] -> w376
            tunnel: w372 -> [w404]
            tunnel: w371 -> [w403]
            frame #0 {
              n209 = feedback #3(u32 0) -> (w394:u32)
              n210 = case shown="False" w397 {
                tunnel: w394 -> [w401 _]
                tunnel: [w401 u32 0] -> w393
                frame False {
                }
                frame True {
                }
              }
              "UDP_Pack_num" <- w393
              n211 = Increment(x=w393) -> (x+1=w395:u32)
              n212 = feedback-in #3(w395) -> ()
            }
            frame #1 {
              n213 = Dequeue Element(queue=w404, error in (no error)=w403) -> (element=w405:string)  [unwired: 1 in, 3 out]
              n214 = UDP Write(address=w408, port or service name=w411, connection ID=w410, data in=w405, 8:w409) -> (error out=w406:errorcluster, 3:w407:refnum<k16>)  [unwired: 1 in]
            }
          }
          n215 = Select(t=FALSE, s=w382, f=TRUE) -> (s? t:f=w379:bool)
          "UDP_Out Status" <- w379
          n216 = local read "stop"() -> (w374:bool)
          n217 = node-c288() -> ()  [unwired: 1 in, 1 out]
          n218 = Unbundle(w376) -> ("status"=w377:bool)  [unwired: 2 out]
          n219 = Compound Arithmetic op=OR(w377, w374) -> (w375:bool)
        }
        n220 = node-c288(w369) -> ()  [unwired: 1 out]
        n221 = UDP Close(connection ID=w362, 8:w361) -> (error out=→"UDP_Out_Error Out":errorcluster)  [unwired: 1 out]
        n222 = Wait (ms)(milliseconds to wait=u32 1000) -> ()  [unwired: 1 out]
      }
      n223 = while {
        tunnel: w61 -> [w79]
        tunnel: w60 -> [w78]
        stop <- w82 stop-if-true
        # "Must Delay to avoid 100% CPU"
        # "TCP Loop writing to FISH Tank"
        n224 = TCP Open Connection(address="192.168.101.110", remote port or service name=u16 3502) -> (connection ID=w85:refnum<k5>, error out=w80:errorcluster)  [unwired: 3 in]
        n225 = case shown="No Error" w80 {
          selector: w80 -> [w90 w117]
          tunnel: w85 -> [w95 w118]
          tunnel: [w94 w118] -> w84
          tunnel: [w93 w117] -> w83
          tunnel: [w92 w116] -> w82
          tunnel: w79 -> [w89 _]
          tunnel: w78 -> [w88 _]
          frame No Error {
            n226 = node-c288() -> (w97:T3)  [unwired: 4 in]
            n227 = timed-loop {
              tunnel: w95 -> [w111]
              tunnel: w90 -> [w110]
              tunnel: [w109] -> w94
              tunnel: [w108] -> w93
              tunnel: [w100] -> w92
              shift-right: [w102] -> _
              shift-left: FALSE -> [w105]
              timing: w97 -> [_]
              timing-out: [_] -> w96
              tunnel: w89 -> [w99]
              tunnel: w88 -> [w98]
              stop <- w106 stop-if-true
              n228 = node-c288() -> ()  [unwired: 1 in, 1 out]
              n229 = Dequeue Element(queue=w99, error in (no error)=w98) -> (element=w101:string)  [unwired: 1 in, 3 out]
              n230 = Select(t=FALSE, s=w105, f=TRUE) -> (s? t:f=w102:bool)
              "TCP packet\nSend To FISH" <- w102
              n231 = TCP Write(connection ID=w111, data in=w101, error in (no error)=w110) -> (connection ID out=w109:refnum<k5>, error out=w108:errorcluster)  [unwired: 1 in, 1 out]
              n232 = local read "stop"() -> (w100:bool)
              n233 = Unbundle(w108) -> ("status"=w107:bool)  [unwired: 2 out]
              n234 = node-c288() -> ()  [unwired: 1 in, 1 out]
              n235 = Compound Arithmetic op=OR(w107, w100) -> (w106:bool)
            }
            n236 = node-c288(w96) -> ()  [unwired: 1 out]
          }
          frame Error {
            n237 = local read "stop"() -> (w116:bool)
          }
        }
        n238 = TCP Close Connection(connection ID=w84, error in (no error)=w83) -> (error out=→"FISH TCP Error Out":errorcluster)  [unwired: 1 in, 1 out]
        n239 = Wait (ms)(milliseconds to wait=u32 1000) -> ()  [unwired: 1 out]
      }
      n240 = node-c288(w46) -> ()  [unwired: 1 out]
      n241 = while {
        tunnel: w63 -> [w121]
        tunnel: w62 -> [w120]
        stop <- w124 stop-if-true
        # "Must Delay to avoid 100% CPU"
        # "TCP Loop writing to SEPTIC Tank"
        n242 = TCP Open Connection(address="192.168.101.108", remote port or service name=u16 3502) -> (connection ID=w127:refnum<k5>, error out=w122:errorcluster)  [unwired: 3 in]
        n243 = case shown="No Error" w122 {
          selector: w122 -> [w132 w159]
          tunnel: w127 -> [w137 w160]
          tunnel: [w136 w160] -> w126
          tunnel: [w135 w159] -> w125
          tunnel: [w134 w158] -> w124
          tunnel: w121 -> [w131 _]
          tunnel: w120 -> [w130 _]
          frame No Error {
            n244 = node-c288() -> (w139:T3)  [unwired: 4 in]
            n245 = timed-loop {
              tunnel: w137 -> [w153]
              tunnel: w132 -> [w152]
              tunnel: [w151] -> w136
              tunnel: [w150] -> w135
              tunnel: [w142] -> w134
              shift-right: [w144] -> _
              shift-left: FALSE -> [w147]
              timing: w139 -> [_]
              timing-out: [_] -> w138
              tunnel: w131 -> [w141]
              tunnel: w130 -> [w140]
              stop <- w148 stop-if-true
              n246 = node-c288() -> ()  [unwired: 1 in, 1 out]
              n247 = Dequeue Element(queue=w141, error in (no error)=w140) -> (element=w143:string)  [unwired: 1 in, 3 out]
              n248 = Select(t=FALSE, s=w147, f=TRUE) -> (s? t:f=w144:bool)
              "TCP packet\nSend To SEPTIC" <- w144
              n249 = TCP Write(connection ID=w153, data in=w143, error in (no error)=w152) -> (connection ID out=w151:refnum<k5>, error out=w150:errorcluster)  [unwired: 1 in, 1 out]
              n250 = local read "stop"() -> (w142:bool)
              n251 = Unbundle(w150) -> ("status"=w149:bool)  [unwired: 2 out]
              n252 = node-c288() -> ()  [unwired: 1 in, 1 out]
              n253 = Compound Arithmetic op=OR(w149, w142) -> (w148:bool)
            }
            n254 = node-c288(w138) -> ()  [unwired: 1 out]
          }
          frame Error {
            n255 = local read "stop"() -> (w158:bool)
          }
        }
        n256 = TCP Close Connection(connection ID=w126, error in (no error)=w125) -> (error out=→"SEPTIC TCP Error Out":errorcluster)  [unwired: 1 in, 1 out]
        n257 = Wait (ms)(milliseconds to wait=u32 1000) -> ()  [unwired: 1 out]
      }
    }
    frame Error {
    }
  }
  n258 = VISA Close(VISA resource name=w25, error in (no error)=w26) -> (error out=→"Serial error out":errorcluster)
